vi "Cannon Angle Calculator.vi"(1 "Distance From Wall":dbl) -> (0 "Needed Angle":dbl)   [LabVIEW 2013]
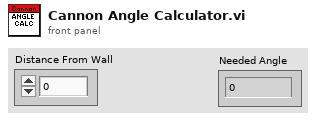
[diagram p1: front panel]
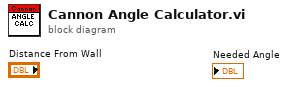
[diagram p0: block diagram]
diagram:
